vi "Read Settings.vi"(8 "error in (no error)":errorcluster, 11 "Neocera LTC-21 in":refnum<class "Neocera LTC-21.lvclass">) -> (0 "error out":errorcluster, 2 "Settings":string, 3 "Neocera LTC-21 out":refnum<class "Neocera LTC-21.lvclass">)   [LabVIEW 2015, in "Neocera LTC-21.lvclass"]
uses:
  Neocera LTC-21.lvclass
  Instrument/Instrument.lvclass
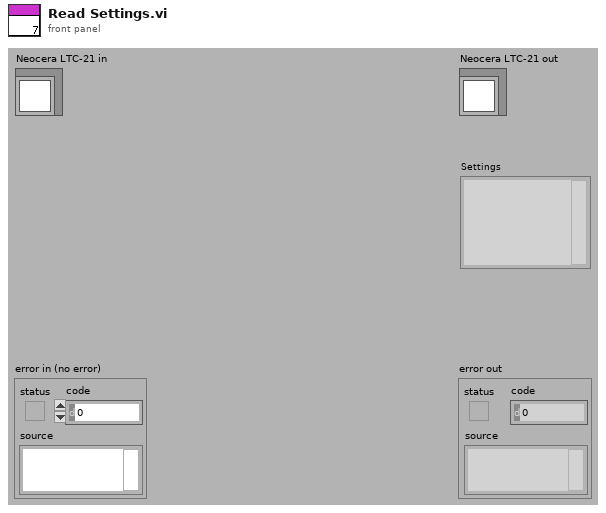
[diagram p1: front panel]
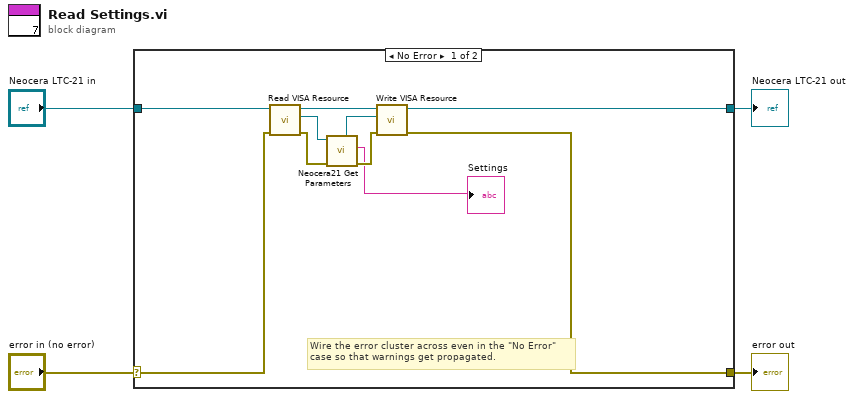
[diagram p0: block diagram]
diagram:
  n1 = case shown="No Error" "error in (no error)" {
    selector: "error in (no error)" -> [w9 w16]
    tunnel: [w6 w16] -> w3
    tunnel: [w12 w15] -> w1
    tunnel: "Neocera LTC-21 in" -> [w13 w15]
    frame No Error {
      # "Wire the error cluster across even in the \"No Error\"\ncase so that warnings get propagated."
      n2 = call "Read VISA Resource.vi"("error in (no error)"=w9, "Instrument.lvclass in"=w13) -> ("error out"=w8:errorcluster, "VISA Resource"=w11:refnum<visa-resource-name>, "Instrument.lvclass out"=w14:refnum<class "Neocera LTC-21.lvclass">)  [unwired: 7 out]
      n3 = call "Neocera21 Get Parameters.vi"("error in (no error)"=w8, "VISA Resource Name"=w11) -> ("error out"=w7:errorcluster, "Parameters"=→"Settings":string, "VISA Resource Name out"=w10:refnum<visa-resource-name>)  [unwired: 1 in, 6 out]
      n4 = call "Write VISA Resource.vi"("error in (no error)"=w7, "VISA Resource"=w10, "Instrument.lvclass in"=w14) -> ("error out"=w6:errorcluster, "Instrument.lvclass out"=w12:refnum<class "Neocera LTC-21.lvclass">)  [unwired: 7 out]
    }
    frame Error {
    }
  }
  "error out" <- w3
  "Neocera LTC-21 out" <- w1
